vi "Flatten Jacobian.vi"(10 "Gradient In":T1[](array[typedef]), 11 "Jacobian":T1[][](array[typedef])) -> (2 "Gradient Out":T1[](array[typedef]))   [LabVIEW 2015, in "Neural Network.lvclass"]
uses:
  Neural Network.lvclass
  Types/2D Array.ctl
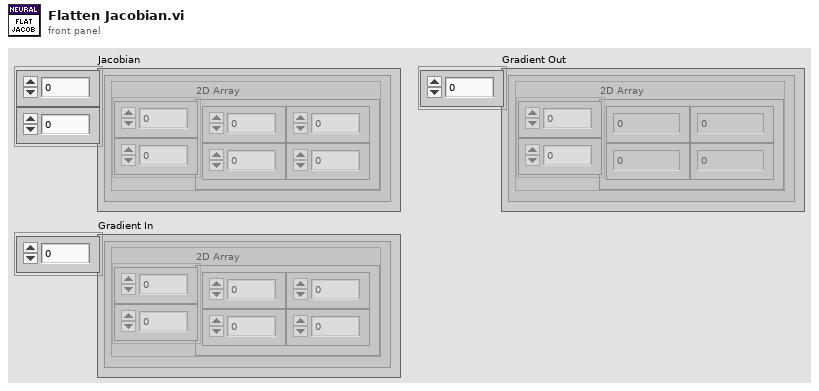
[diagram p1: front panel]
types:
  T1 = typedef "Neural Network.lvclass/2D Array.ctl" = cluster{"2D Array":sgl[][]}
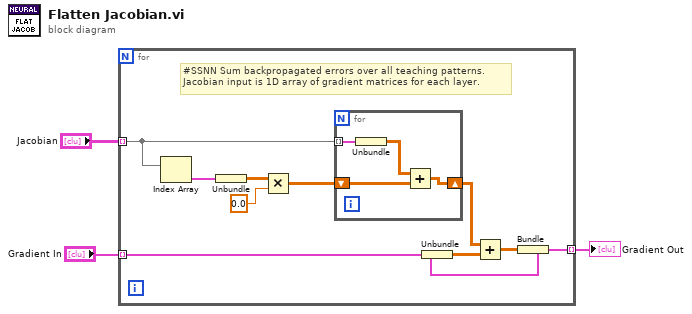
[diagram p0: block diagram]
diagram:
  n1 = for {
    tunnel: "Jacobian" -> [w8] mode=indexing
    tunnel: [w13] -> w1 mode=indexing
    tunnel: "Gradient In" -> [w4] mode=indexing
    # "#SSNN Sum backpropagated errors over all teaching patterns.\nJacobian input is 1D array of gradient matrices for each layer."
    n2 = Index Array(array=w8) -> (element=w12:T1)  [unwired: 1 in]
    n3 = Unbundle(w12) -> ("2D Array"=w11:sgl[][])
    n4 = Multiply(x=w11, y=0.0) -> (x*y=w9:dbl[][])
    n5 = for {
      tunnel: w8 -> [w17] mode=indexing
      shift-right: [w14] -> w6
      shift-left: w9 -> [w16]
      n6 = Unbundle(w17) -> ("2D Array"=w15:sgl[][])
      n7 = Add(x=w15, y=w16) -> (x+y=w14:dbl[][])
    }
    n8 = Unbundle(w4) -> ("2D Array"=w7:sgl[][])
    n9 = Add(x=w6, y=w7) -> (x+y=w5:dbl[][])
    n10 = Bundle(cluster=w4, "2D Array"=w5) -> (w13:T1)
  }
  "Gradient Out" <- w1
